vi "reading_data_from_files.vi"() -> (0 "Super_Heated_T_Curves":T1, 1 "Super_Heated_S_Curves":T2, 2 "Sat_Deg_10_Step":T3, 3 "Sat_By_Deg":T4)   [LabVIEW 2017]
uses:
  <vilib>/Utility/error.llb/DialogType.ctl
  <vilib>/Utility/file.llb/Read Delimited Spreadsheet (DBL).vi
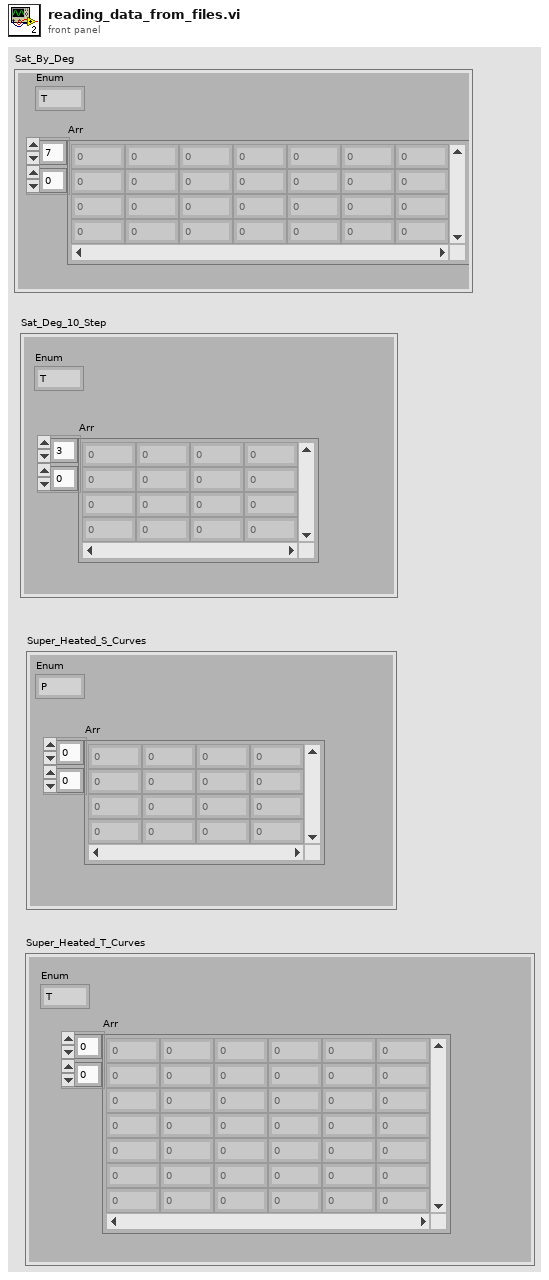
[diagram p1: front panel]
types:
  T1 = cluster{"Enum":enum16{"T", "P", "T_Sat_Vapor", "Hg", "Sg", "Vg"}, "Arr":dbl[][]}
  T2 = cluster{"Enum":enum16{"P", "S", "H gas"}, "Arr":dbl[][]}
  T3 = cluster{"Enum":enum16{"T", "P", "V1", "Vg", "H1", "Hg", "R", "S1", "Sg"}, "Arr":dbl[][]}
  T4 = cluster{"Enum":enum16{"T", "P", "V1", "Vg", "H1", "Hg", "R", "S1", "Sg"}, "Arr ":dbl[][]}
  T5 = typedef "DialogType.ctl" = u16
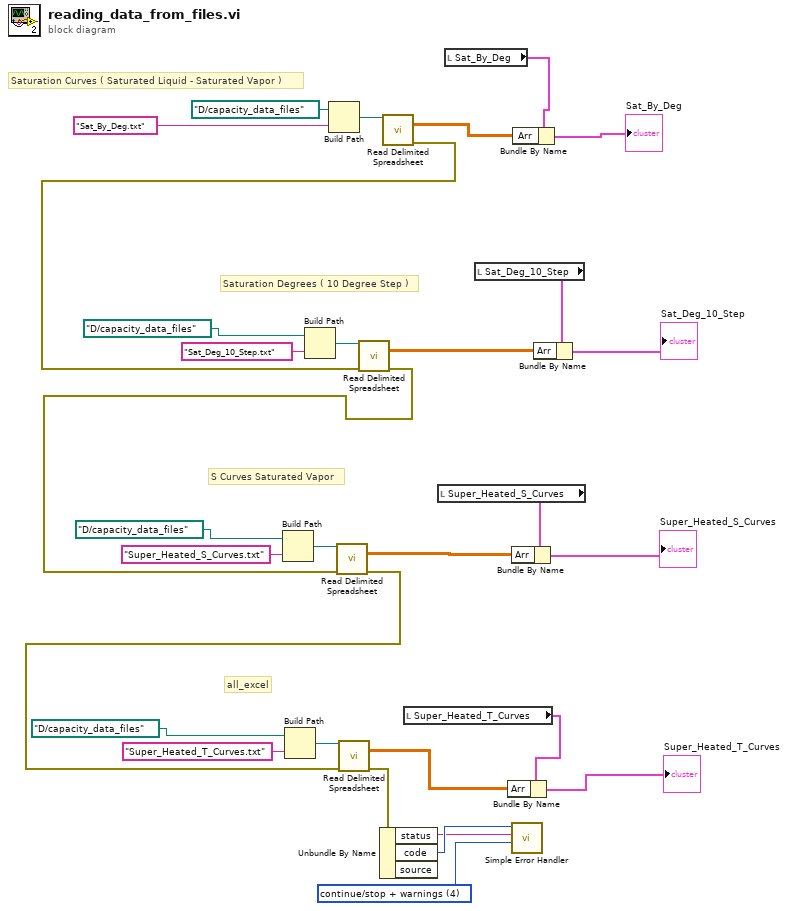
[diagram p0: block diagram]
diagram:
  w9 = T5 4 items=["no dialog", "OK message", "continue or stop message", "OK message + warnings", "continue/stop + warnings"] ("type of dialog (OK msg:1)")
  # "all_excel"
  # "S Curves Saturated Vapor"
  # "Saturation Curves ( Saturated Liquid - Saturated Vapor )"
  # "Saturation Degrees ( 10 Degree Step )"
  n1 = Build Path(base path=path "D:/capacity_data_files", name or relative path="Super_Heated_S_Curves.txt") -> (appended path=w31:path)
  n2 = Build Path(base path=path "D:/capacity_data_files", name or relative path="Super_Heated_T_Curves.txt") -> (appended path=w28:path)
  n3 = Build Path(base path=path "D:/capacity_data_files", name or relative path="Sat_Deg_10_Step.txt") -> (appended path=w25:path)
  n4 = Build Path(base path=path "D:/capacity_data_files", name or relative path="Sat_By_Deg.txt") -> (appended path=w30:path)
  n5 = call-poly <vilib>:"Read Delimited Spreadsheet.vi"("file path (dialog if empty)"=w30) -> ("all rows"=w23:dbl[][], "error out"=w2:errorcluster)  [unwired: 9 in, 4 out]
  n6 = call-poly <vilib>:"Read Delimited Spreadsheet.vi"("file path (dialog if empty)"=w25, "error in (no error)"=w2) -> ("all rows"=w21:dbl[][], "error out"=w3:errorcluster)  [unwired: 8 in, 4 out]
  n7 = call-poly <vilib>:"Read Delimited Spreadsheet.vi"("file path (dialog if empty)"=w31, "error in (no error)"=w3) -> ("all rows"=w19:dbl[][], "error out"=w1:errorcluster)  [unwired: 8 in, 4 out]
  n8 = call-poly <vilib>:"Read Delimited Spreadsheet.vi"("file path (dialog if empty)"=w28, "error in (no error)"=w1) -> ("all rows"=w18:dbl[][], "error out"=w8:errorcluster)  [unwired: 8 in, 4 out]
  n9 = Unbundle By Name(w8) -> ("code"=w11:i32, "source"=w10:string)  [unwired: 1 out]
  n10 = local read "Super_Heated_T_Curves"() -> (w12:T1)
  n11 = local read "Super_Heated_S_Curves"() -> (w13:T2)
  n12 = local read "Sat_By_Deg"() -> (w15:T4)
  n13 = local read "Sat_Deg_10_Step"() -> (w14:T3)
  n14 = Bundle By Name(cluster=w12, "Arr"=w18) -> (→"Super_Heated_T_Curves":T1)
  n15 = Bundle By Name(cluster=w13, "Arr"=w19) -> (→"Super_Heated_S_Curves":T2)
  n16 = call <vilib>:"Simple Error Handler.vi"("error code (no error:0)"=w11, "error source (\" \")"=w10, "type of dialog (OK msg:1)"=w9) -> ()  [unwired: 2 in, 5 out]
  n17 = Bundle By Name(cluster=w15, "Arr"=w23) -> (→"Sat_By_Deg":T4)
  n18 = Bundle By Name(cluster=w14, "Arr"=w21) -> (→"Sat_Deg_10_Step":T3)
